vi "Periodic Tasks.vi"(8 "error in":errorcluster) -> ()   [LabVIEW 2013]
doc: "This VI runs in parallel to other tasks. It can contain as many user-defined periodic loops as you need. These can carry out PID or other sorts of timed response."
uses:
  <vilib>/Rock Robotics/SystemInterfaces/Utilities/FPGA_UtilitiesLED Source.ctl
  <vilib>/Rock Robotics/SystemInterfaces/Utilities/FPGA_UtilitiesLED State.ctl
  Robot Global Data.vi
  <vilib>/Rock Robotics/WPI/Joystick/WPI_JoystickGetSetRefNum.vi
panel:
  out "Claw esquerda":dbl
  out "Claw direita":dbl
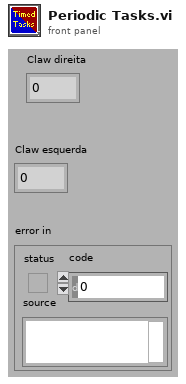
[diagram p1: front panel]
types:
  T1 = typedef "WPI_JoystickDevRef.ctl" = cluster{"Device":T2}
  T2 = typedef "WPI_JoystickDeviceEnum.ctl" = enum16{"USB 1", "USB 2", "USB 3", "USB 4", "Kinect 1", "Kinect 2"}
  T3 = typedef "WPI_DigitalInputDevRef.ctl" = cluster{"DevStatus":errorcluster, "DIO Channel":T4, "Digital Module":T5}
  T4 = typedef "FPGA_DIOChannel.ctl" = enum8{"DIO 1", "DIO 2", "DIO 3", "DIO 4", "DIO 5", "DIO 6", "DIO 7", "DIO 8", "DIO 9", "DIO 10", "DIO 11", "DIO 12", "DIO 13", "DIO 14", "Invalid"}
  T5 = typedef "FPGA_TypedefDigitalModule.ctl" = enum16{"Digital Module 1", "Digital Module 2"}
  T6 = typedef "WPI_JoystickButtonState.ctl" = cluster{"Button 1":bool, "Button 2":bool, "Button 3":bool, "Button 4":bool, "Button 5":bool, "Button 6":bool, "Button 7":bool, "Button 8":bool, "Button 9":bool, "Button 10":bool, "Button 11":bool, "Button 12":bool}
  T7 = typedef "WPI_MotorControlDeviceRef.ctl" = cluster{"DeviceStatus":errorcluster, "Type":enum16{"PWM", "CAN"}, "PWM":cluster{"Digital Module":T5, "PWM Channel":T8, "DeadBand":T9}, "CAN":cluster{"Device Number":u8, "Control Mode":T10, "Semaphore":T11, "Max Vout":dbl}, "Invert":bool, "TransformRef":T12, "InvTransformRef":T12}
  T8 = typedef "FPGA_DIOPWMChannel.ctl" = enum8{"PWM 1", "PWM 2", "PWM 3", "PWM 4", "PWM 5", "PWM 6", "PWM 7", "PWM 8", "PWM 9", "PWM 10", "Invalid"}
  T9 = typedef "WPI_PWMDeadband.ctl" = cluster{"Name":string, "maxPositivePwm":i32, "minPositivePwm":i32, "centerPwm":i32, "maxNegativePwm":i32, "minNegativePwm":i32, "angularRange":u16}
  T10 = typedef "WPI_CANJaguar_ControlMode.ctl" = enum8{"Percent VBus", "Current", "Speed", "Position", "Voltage"}
  T11 = typedef "Semaphore RefNum" = refnum<k1>
  T12 = typedef "WPI_PWMTransform_ConPane.ctl" = refnum<vi>
  T13 = typedef "WPI_DriverStationRobotMode2.ctl" = enum16{"Autonomous Disabled", "Autonomous Enabled", "Teleop Disabled", "Teleop Enabled", "Timeout", "Finish", "Test Disabled", "Test Enabled"}
  T14 = typedef "WPI_ServoDeviceRef.ctl" = cluster{"DeviceStatus":errorcluster, "Digital Module":T5, "PWM Channel":T8, "DeadBand":T9}
  T15 = cluster{"axis 1 (x)":dbl, "axis 2 (y)":dbl, "axis 3 (throttle)":dbl, "axis 4":dbl, "axis 5":dbl, "axis 6":dbl}
  T16 = typedef "FPGA_UtilitiesLED State.ctl" = enum16{"Off", "On", "Toggle"}
  T17 = typedef "FPGA_UtilitiesLED Source.ctl" = enum16{"User LED", "FPGA LED"}
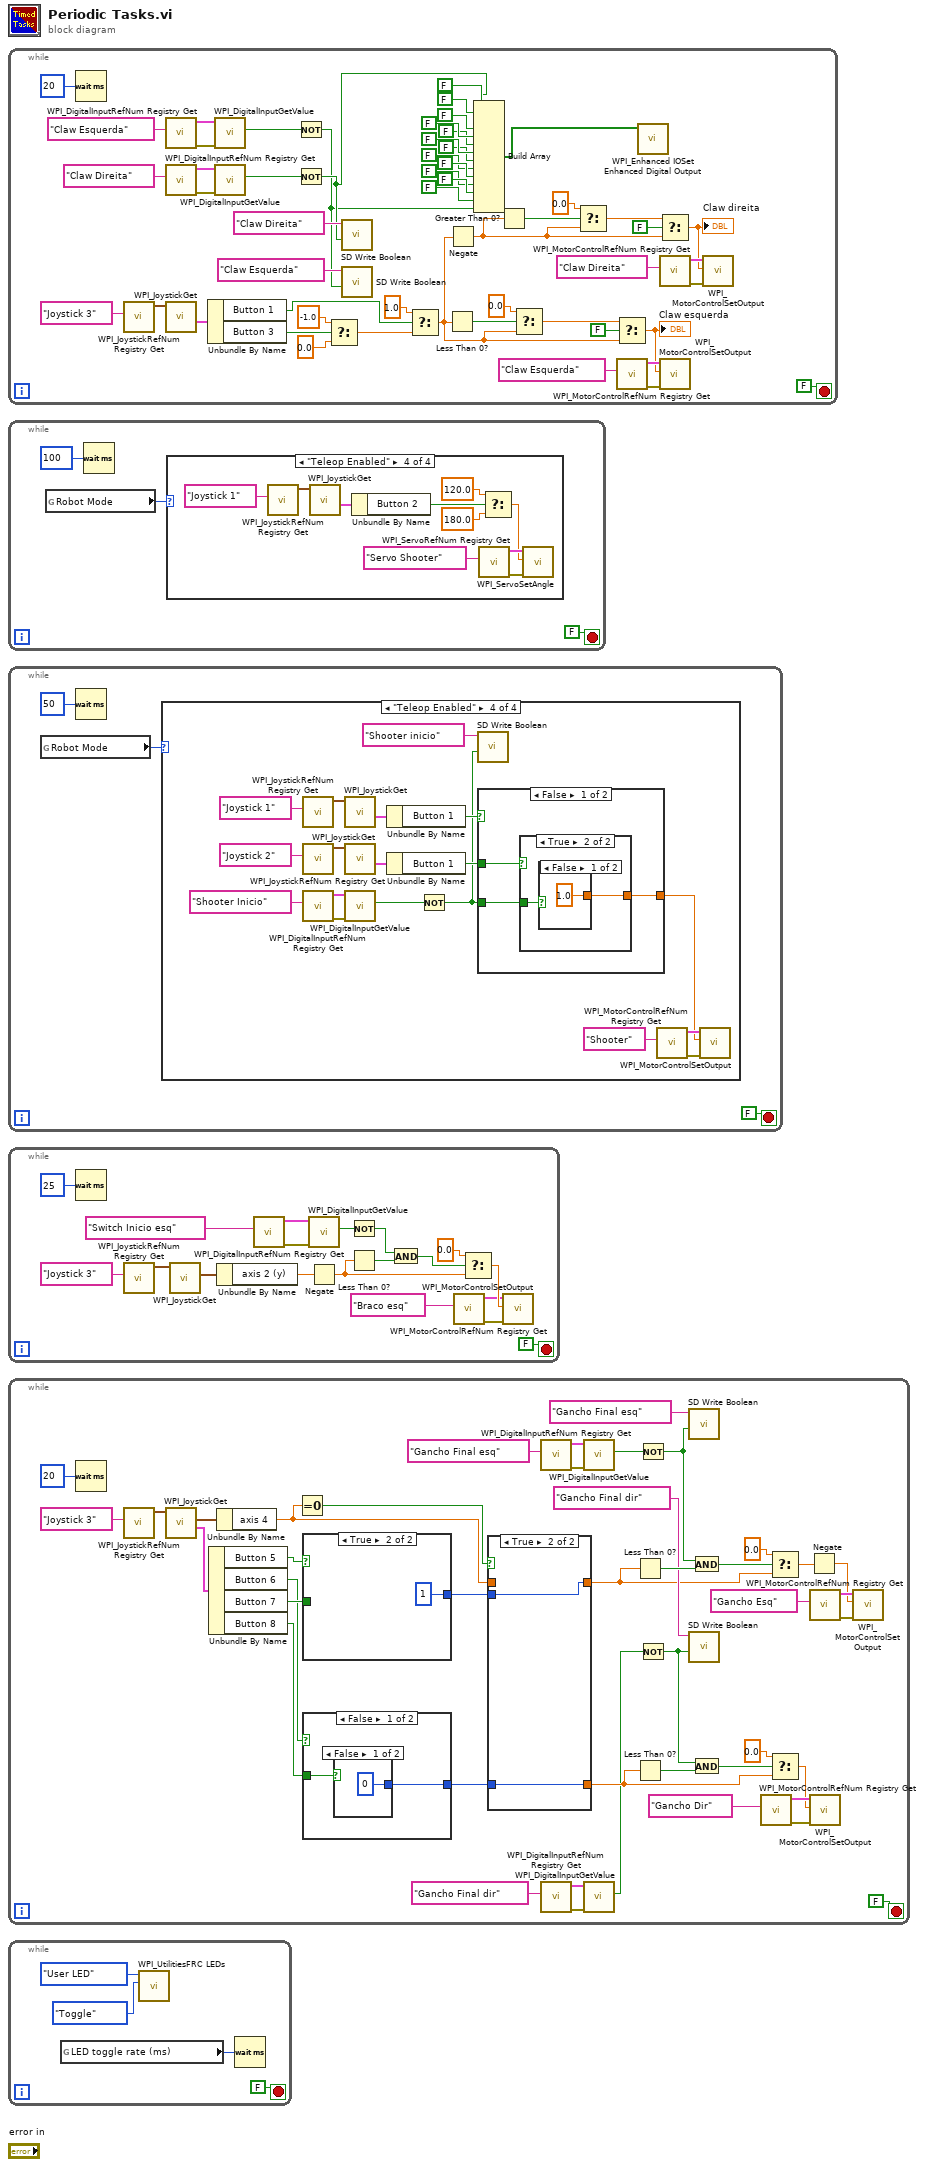
[diagram p0: block diagram]
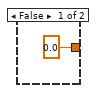
[diagram p8: hidden frame]
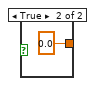
[diagram p9: hidden frame]
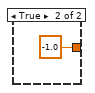
[diagram p10: hidden frame]
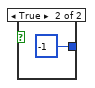
[diagram p11: hidden frame]
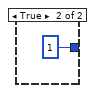
[diagram p12: hidden frame]
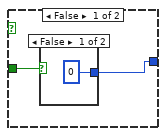
[diagram p13: hidden frame]
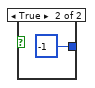
[diagram p14: hidden frame]
diagram:
  n1 = while {
    stop <- FALSE stop-if-true
    n2 = Wait (ms)(milliseconds to wait=u32 20) -> ()  [unwired: 1 out]
    n3 = call <vilib>:"WPI_JoystickRefNum Registry Get.vi"("refnum name"="Joystick 3") -> ("JoystickDevRef"=w44:T1)  [unwired: 9 in, 1 out]
    n4 = call <vilib>:"WPI_DigitalInputRefNum Registry Get.vi"("refnum name"="Claw Esquerda") -> ("error out"=w47:errorcluster, "DigitalInputDevRef"=w46:T3)  [unwired: 9 in]
    n5 = call <vilib>:"WPI_DigitalInputRefNum Registry Get.vi"("refnum name"="Claw Direita") -> ("error out"=w52:errorcluster, "DigitalInputDevRef"=w51:T3)  [unwired: 9 in]
    n6 = call <vilib>:"WPI_JoystickGet.vi"("JoystickDevRef"=w44) -> ("Buttons"=w37:T6)  [unwired: 4 in, 2 out]
    n7 = Unbundle By Name(w37) -> ("Button 1"=w22:bool, "Button 3"=w21:bool)
    n8 = call <vilib>:"WPI_DigitalInputGetValue.vi"("error in (no error)"=w47, "DigitalInputDevRef"=w46) -> ("Value"=w35:bool)  [unwired: 7 in, 2 out]
    n9 = call <vilib>:"WPI_DigitalInputGetValue.vi"("error in (no error)"=w52, "DigitalInputDevRef"=w51) -> ("Value"=w36:bool)  [unwired: 7 in, 2 out]
    n10 = Not(x=w35) -> (.not. x?=w2:bool)
    n11 = Not(x=w36) -> (.not. x?=w3:bool)
    n12 = Select(t=-1.0, s=w21, f=0.0) -> (s? t:f=w24:dbl)
    n13 = call <vilib>:"SD Write Boolean.vi"("Boolean"=w3, "Name"="Claw Direita") -> ()  [unwired: 8 in, 2 out]
    n14 = call <vilib>:"SD Write Boolean.vi"("Boolean"=w2, "Name"="Claw Esquerda") -> ()  [unwired: 8 in, 2 out]
    n15 = Select(t=1.0, s=w22, f=w24) -> (s? t:f=w33:dbl)
    n16 = Less Than 0?(x=w33) -> (x < 0?=w32:bool)
    n17 = Negate(x=w33) -> (-x=w29:dbl)
    n18 = Build Array(w3, FALSE ("element"), FALSE ("element"), FALSE ("element"), FALSE ("element"), FALSE ("element"), FALSE ("element"), FALSE ("element"), FALSE ("element"), FALSE ("element"), FALSE ("element"), FALSE ("element"), FALSE ("element"), w2) -> (w1:bool[])
    n19 = Greater Than 0?(x=w29) -> (x > 0?=w27:bool)
    n20 = Select(t=0.0, s=w32, f=w33) -> (s? t:f=w30:dbl)
    n21 = Select(t=0.0, s=w27, f=w29) -> (s? t:f=w26:dbl)
    n22 = Select(t=w30, s=FALSE, f=w33) -> (s? t:f=w19:dbl)
    "Claw esquerda" <- w19
    n23 = call <vilib>:"WPI_MotorControlRefNum Registry Get.vi"("refnum name"="Claw Esquerda") -> ("error out"=w48:errorcluster, "MotorControlDevRef"=w45:T7)  [unwired: 9 in]
    n24 = call <vilib>:"WPI_Enhanced IOSet Enhanced Digital Output.vi"("Digital Output [1-16]"=w1) -> ()  [unwired: 10 in, 1 out]
    n25 = Select(t=w26, s=FALSE, f=w29) -> (s? t:f=w20:dbl)
    "Claw direita" <- w20
    n26 = call <vilib>:"WPI_MotorControlRefNum Registry Get.vi"("refnum name"="Claw Direita") -> ("error out"=w39:errorcluster, "MotorControlDevRef"=w40:T7)  [unwired: 9 in]
    n27 = call <vilib>:"WPI_MotorControlSetOutput.vi"("error in (no error)"=w48, "Output"=w19, "MotorControlDevRef"=w45) -> ()  [unwired: 6 in, 3 out]
    n28 = call <vilib>:"WPI_MotorControlSetOutput.vi"("error in (no error)"=w39, "Output"=w20, "MotorControlDevRef"=w40) -> ()  [unwired: 6 in, 3 out]
  }
  n29 = while {
    stop <- FALSE stop-if-true
    n30 = global read "Robot Global Data.vi" "Robot Mode"() -> (w55:T13)
    n31 = Wait (ms)(milliseconds to wait=u32 100) -> ()  [unwired: 1 out]
    n32 = case shown="\"Teleop Enabled\"" w55 {
      frame "Autonomous Disabled", Default {
      }
      frame "Autonomous Enabled" {
      }
      frame "Teleop Disabled" {
      }
      frame "Teleop Enabled" {
        n33 = call <vilib>:"WPI_JoystickRefNum Registry Get.vi"("refnum name"="Joystick 1") -> ("JoystickDevRef"=w63:T1)  [unwired: 9 in, 1 out]
        n34 = call <vilib>:"WPI_JoystickGet.vi"("JoystickDevRef"=w63) -> ("Buttons"=w62:T6)  [unwired: 4 in, 2 out]
        n35 = Unbundle By Name(w62) -> ("Button 2"=w58:bool)
        n36 = call <vilib>:"WPI_ServoRefNum Registry Get.vi"("refnum name"="Servo Shooter") -> ("error out"=w67:errorcluster, "ServoDeviceRef"=w66:T14)  [unwired: 9 in]
        n37 = Select(t=120.0, s=w58, f=180.0) -> (s? t:f=w61:dbl)
        n38 = call <vilib>:"WPI_ServoSetAngle.vi"("error in (no error)"=w67, "Angle"=w61, "ServoDeviceRef"=w66) -> ()  [unwired: 7 in, 2 out]
      }
    }
  }
  n39 = while {
    stop <- FALSE stop-if-true
    n40 = global read "Robot Global Data.vi" "Robot Mode"() -> (w68:T13)
    n41 = Wait (ms)(milliseconds to wait=u32 50) -> ()  [unwired: 1 out]
    n42 = case shown="\"Teleop Enabled\"" w68 {
      frame "Autonomous Disabled", Default {
      }
      frame "Autonomous Enabled" {
      }
      frame "Teleop Disabled" {
      }
      frame "Teleop Enabled" {
        n43 = call <vilib>:"WPI_JoystickRefNum Registry Get.vi"("refnum name"="Joystick 1") -> ("JoystickDevRef"=w86:T1)  [unwired: 9 in, 1 out]
        n44 = call <vilib>:"WPI_JoystickRefNum Registry Get.vi"("refnum name"="Joystick 2") -> ("JoystickDevRef"=w79:T1)  [unwired: 9 in, 1 out]
        n45 = call <vilib>:"WPI_DigitalInputRefNum Registry Get.vi"("refnum name"="Shooter Inicio") -> ("error out"=w82:errorcluster, "DigitalInputDevRef"=w83:T3)  [unwired: 9 in]
        n46 = call <vilib>:"WPI_JoystickGet.vi"("JoystickDevRef"=w86) -> ("Buttons"=w76:T6)  [unwired: 4 in, 2 out]
        n47 = call <vilib>:"WPI_JoystickGet.vi"("JoystickDevRef"=w79) -> ("Buttons"=w77:T6)  [unwired: 4 in, 2 out]
        n48 = call <vilib>:"WPI_DigitalInputGetValue.vi"("error in (no error)"=w82, "DigitalInputDevRef"=w83) -> ("Value"=w72:bool)  [unwired: 7 in, 2 out]
        n49 = Unbundle By Name(w76) -> ("Button 1"=w75:bool)
        n50 = Unbundle By Name(w77) -> ("Button 1"=w73:bool)
        n51 = Not(x=w72) -> (.not. x?=w71:bool)
        n52 = call <vilib>:"SD Write Boolean.vi"("Boolean"=w71, "Name"="Shooter inicio") -> ()  [unwired: 8 in, 2 out]
        n53 = case shown="False" w75 {
          tunnel: [w89 -1.0 ("Output")] -> w74
          tunnel: w73 -> [w91 _]
          tunnel: w71 -> [w90 _]
          frame False {
            n54 = case shown="True" w91 {
              tunnel: w90 -> [_ w94]
              tunnel: [0.0 ("Output") w93] -> w89
              frame False {
              }
              frame True {
                n55 = case shown="False" w94 {
                  tunnel: [1.0 ("Output") 0.0 ("Output")] -> w93
                  frame False {
                  }
                  frame True {
                  }
                }
              }
            }
          }
          frame True {
          }
        }
        n56 = call <vilib>:"WPI_MotorControlRefNum Registry Get.vi"("refnum name"="Shooter") -> ("error out"=w84:errorcluster, "MotorControlDevRef"=w85:T7)  [unwired: 9 in]
        n57 = call <vilib>:"WPI_MotorControlSetOutput.vi"("error in (no error)"=w84, "Output"=w74, "MotorControlDevRef"=w85) -> ()  [unwired: 6 in, 3 out]
      }
    }
  }
  n58 = while {
    stop <- FALSE stop-if-true
    n59 = Wait (ms)(milliseconds to wait=u32 25) -> ()  [unwired: 1 out]
    n60 = call <vilib>:"WPI_JoystickRefNum Registry Get.vi"("refnum name"="Joystick 3") -> ("JoystickDevRef"=w114:T1)  [unwired: 9 in, 1 out]
    n61 = call <vilib>:"WPI_JoystickGet.vi"("JoystickDevRef"=w114) -> ("Axes"=w107:T15)  [unwired: 4 in, 2 out]
    n62 = Unbundle By Name(w107) -> ("axis 2 (y)"=w103:dbl)
    n63 = call <vilib>:"WPI_DigitalInputRefNum Registry Get.vi"("refnum name"="Switch Inicio esq") -> ("error out"=w112:errorcluster, "DigitalInputDevRef"=w111:T3)  [unwired: 9 in]
    n64 = call <vilib>:"WPI_DigitalInputGetValue.vi"("error in (no error)"=w112, "DigitalInputDevRef"=w111) -> ("Value"=w109:bool)  [unwired: 7 in, 2 out]
    n65 = Negate(x=w103) -> (-x=w98:dbl)
    n66 = Not(x=w109) -> (.not. x?=w108:bool)
    n67 = Less Than 0?(x=w98) -> (x < 0?=w106:bool)
    n68 = And(x=w108, y=w106) -> (x .and. y?=w105:bool)
    n69 = call <vilib>:"WPI_MotorControlRefNum Registry Get.vi"("refnum name"="Braco esq") -> ("error out"=w101:errorcluster, "MotorControlDevRef"=w100:T7)  [unwired: 9 in]
    n70 = Select(t=0.0, s=w105, f=w98) -> (s? t:f=w102:dbl)
    n71 = call <vilib>:"WPI_MotorControlSetOutput.vi"("error in (no error)"=w101, "Output"=w102, "MotorControlDevRef"=w100) -> ()  [unwired: 6 in, 3 out]
  }
  n72 = while {
    stop <- FALSE stop-if-true
    n73 = Wait (ms)(milliseconds to wait=u32 20) -> ()  [unwired: 1 out]
    n74 = call <vilib>:"WPI_JoystickRefNum Registry Get.vi"("refnum name"="Joystick 3") -> ("JoystickDevRef"=w154:T1)  [unwired: 9 in, 1 out]
    n75 = call <vilib>:"WPI_JoystickGet.vi"("JoystickDevRef"=w154) -> ("Buttons"=w123:T6, "Axes"=w133:T15)  [unwired: 4 in, 1 out]
    n76 = Unbundle By Name(w123) -> ("Button 5"=w122:bool, "Button 6"=w119:bool, "Button 7"=w120:bool, "Button 8"=w117:bool)
    n77 = Unbundle By Name(w133) -> ("axis 4"=w130:dbl)
    n78 = Equal To 0?(x=w130) -> (x = 0?=w131:bool)
    n79 = case shown="True" w122 {
      tunnel: w120 -> [w166 _]
      tunnel: [w165 1] -> w121
      frame False {
        n80 = case shown="False" w166 {
          tunnel: [0 -1] -> w165
          frame False {
          }
          frame True {
          }
        }
      }
      frame True {
      }
    }
    n81 = case shown="False" w119 {
      tunnel: [w161 1] -> w118
      tunnel: w117 -> [w160 _]
      frame False {
        n82 = case shown="False" w160 {
          tunnel: [0 -1] -> w161
          frame False {
          }
          frame True {
          }
        }
      }
      frame True {
      }
    }
    n83 = case shown="True" w131 {
      tunnel: [w170 w171] -> w128
      tunnel: [w170 w172] -> w129
      tunnel: w121 -> [_ w172]
      tunnel: w130 -> [w170 _]
      tunnel: w118 -> [_ w171]
      frame False {
      }
      frame True {
      }
    }
    n84 = call <vilib>:"WPI_DigitalInputRefNum Registry Get.vi"("refnum name"="Gancho Final esq") -> ("error out"=w148:errorcluster, "DigitalInputDevRef"=w147:T3)  [unwired: 9 in]
    n85 = call <vilib>:"WPI_DigitalInputRefNum Registry Get.vi"("refnum name"="Gancho Final dir") -> ("error out"=w149:errorcluster, "DigitalInputDevRef"=w150:T3)  [unwired: 9 in]
    n86 = call <vilib>:"WPI_DigitalInputGetValue.vi"("error in (no error)"=w148, "DigitalInputDevRef"=w147) -> ("Value"=w127:bool)  [unwired: 7 in, 2 out]
    n87 = call <vilib>:"WPI_DigitalInputGetValue.vi"("error in (no error)"=w149, "DigitalInputDevRef"=w150) -> ("Value"=w126:bool)  [unwired: 7 in, 2 out]
    n88 = Less Than 0?(x=w129) -> (x < 0?=w139:bool)
    n89 = Less Than 0?(x=w128) -> (x < 0?=w144:bool)
    n90 = Not(x=w127) -> (.not. x?=w125:bool)
    n91 = Not(x=w126) -> (.not. x?=w124:bool)
    n92 = call <vilib>:"SD Write Boolean.vi"("Boolean"=w125, "Name"="Gancho Final esq") -> ()  [unwired: 8 in, 2 out]
    n93 = call <vilib>:"SD Write Boolean.vi"("Boolean"=w124, "Name"="Gancho Final dir") -> ()  [unwired: 8 in, 2 out]
    n94 = And(x=w125, y=w139) -> (x .and. y?=w140:bool)
    n95 = And(x=w124, y=w144) -> (x .and. y?=w143:bool)
    n96 = call <vilib>:"WPI_MotorControlRefNum Registry Get.vi"("refnum name"="Gancho Dir") -> ("error out"=w157:errorcluster, "MotorControlDevRef"=w158:T7)  [unwired: 9 in]
    n97 = Select(t=0.0, s=w140, f=w129) -> (s? t:f=w137:dbl)
    n98 = Select(t=0.0, s=w143, f=w128) -> (s? t:f=w141:dbl)
    n99 = Negate(x=w137) -> (-x=w132:dbl)
    n100 = call <vilib>:"WPI_MotorControlRefNum Registry Get.vi"("refnum name"="Gancho Esq") -> ("error out"=w153:errorcluster, "MotorControlDevRef"=w151:T7)  [unwired: 9 in]
    n101 = call <vilib>:"WPI_MotorControlSetOutput.vi"("error in (no error)"=w157, "Output"=w141, "MotorControlDevRef"=w158) -> ()  [unwired: 6 in, 3 out]
    n102 = call <vilib>:"WPI_MotorControlSetOutput.vi"("error in (no error)"=w153, "Output"=w132, "MotorControlDevRef"=w151) -> ()  [unwired: 6 in, 3 out]
  }
  n103 = while {
    stop <- FALSE stop-if-true
    n104 = global read "Robot Global Data.vi" "LED toggle rate (ms)"() -> (w173:u32)
    n105 = call <vilib>:"WPI_UtilitiesFRC LEDs.vi"("State"=FPGA_UtilitiesLED_State."Toggle", "LED Type"=FPGA_UtilitiesLED_Source."User LED") -> ()  [unwired: 1 in, 9 out]
    n106 = Wait (ms)(milliseconds to wait=w173) -> ()  [unwired: 1 out]
  }
